vi "Read Measurement (Spurious Emission).vi"(0 "VISA resource name":refnum<visa-resource-name>, 11 "error in (no error)":errorcluster) -> (4 "VISA resource name out":refnum<visa-resource-name>, 6 "Judgement Result":i32(ring) items=["PASS", "FAIL"], 8 "Data Count":i32, 10 "Spurious Emission":T1(array[cluster]) {"Judgement" items=["PASS", "FAIL"]; "Peark" format="%.2f"; "Margin" format="%.3f"; "Limit" format="%.2f"}, 15 "error out":errorcluster)   [LabVIEW 2020, in "Anritsu Signal Analyzer Series.lvlib"]
doc: "Reads Spurious Emission measurement Data"
uses:
  Anritsu Signal Analyzer Series.lvlib
panel:
  # "Judgement"
  # "No."
  # "Segment"
  # "Frequency(Hz)"
  # "Peak(dBm)"
  # "Margin(dB)"
  # "Limit(dBm)"
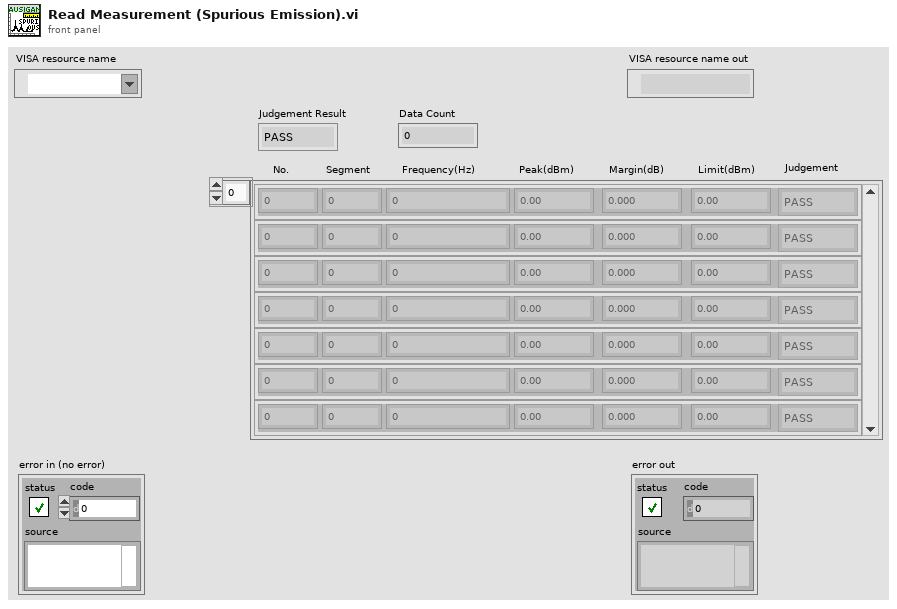
[diagram p1: front panel]
types:
  T1 = cluster{"No.":dbl, "Segment":dbl, "Frequency":dbl, "Peark":dbl, "Margin":dbl, "Limit":dbl, "Judgement":i32}[]
  T2 = cluster{"Numeric":dbl, "Numeric":dbl, "Numeric":dbl, "Numeric":dbl, "Numeric":dbl, "Numeric":dbl, "Numeric":dbl}
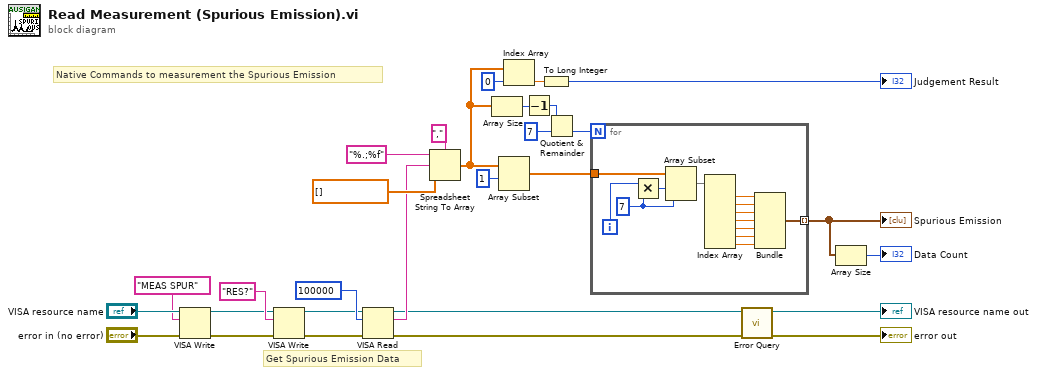
[diagram p0: block diagram]
diagram:
  # "Native Commands to measurement the Spurious Emission"
  # "Get Spurious Emission Data"
  n1 = VISA Write(VISA resource name="VISA resource name", write buffer="MEAS SPUR" ("_CommandSet"), error in (no error)="error in (no error)") -> (VISA resource name out=w2:refnum<visa-resource-name>, error out=w1:errorcluster)  [unwired: 1 out]
  n2 = VISA Write(VISA resource name=w2, write buffer="RES?" ("_Command"), error in (no error)=w1) -> (VISA resource name out=w9:refnum<visa-resource-name>, error out=w7:errorcluster)  [unwired: 1 out]
  n3 = VISA Read(VISA resource name=w9, byte count=u32 100000 ("byte count (0)"), error in (no error)=w7) -> (VISA resource name out=w5:refnum<visa-resource-name>, read buffer=w13:string, error out=w6:errorcluster)  [unwired: 1 out]
  n4 = Spreadsheet String To Array(delimiter (Tab)=",", format string="%.;%f", spreadsheet string=w13, array type (2D Dbl)=dbl[] [] ("Values")) -> (array=w8:dbl[])
  n5 = Array Size(array=w8) -> (size(s)=w21:i32)
  n6 = Array Subset(array=w8, index=1 ("Žw•W")) -> (w17:dbl[])  [unwired: 1 in]
  n7 = Index Array(array=w8, index=0 ("Žw•W")) -> (element=w15:dbl)
  n8 = Decrement(x=w21) -> (x-1=w20:i32)
  n9 = To Long Integer(number=w15) -> (32bit integer=→"Judgement Result":i32)
  n10 = Quotient & Remainder(x=w20, y=7) -> (floor(x/y)=w18:i32)  [unwired: 1 out]
  n11 = for {
    N: w18 -> [_]
    tunnel: w17 -> [w42]
    tunnel: [w32] -> w26 mode=indexing
    i -> [w41]
    w39 = 7 ("y")
    n12 = Multiply(x=w41, y=w39) -> (x*y=w40:i32)
    n13 = Array Subset(array=w42, index=w40, length=w39) -> (w38:dbl[])
    n14 = Index Array(array=w38) -> (element #1=w37:dbl, element #2=w36:dbl, element #3=w31:dbl, element #4=w35:dbl, element #5=w34:dbl, element #6=w33:dbl, element #7=w30:dbl)  [unwired: 7 in]
    n15 = Bundle("Numeric"=w37, "Numeric"=w36, "Numeric"=w31, "Numeric"=w35, "Numeric"=w34, "Numeric"=w33, "Numeric"=w30) -> (w32:T2)  [unwired: 1 in]
  }
  "Spurious Emission" <- w26
  n16 = call "Error Query.vi"("error in (no error)"=w6, "VISA resource name"=w5) -> ("error out"=→"error out":errorcluster, "VISA resource name out"=→"VISA resource name out":refnum<visa-resource-name>)  [unwired: 6 in, 2 out]
  n17 = Array Size(array=w26) -> (size(s)=→"Data Count":i32)
